vi "Set Position.vi"(0 "LV MDI.lvclass":refnum<class "LV MDI.lvclass">, 5 "Doc UID[]":string[](array[string]), 7 "Position[]":T1[](array[typedef]), 11 "error in (no error)":errorcluster) -> (4 "LV MDI.lvclass":refnum<class "LV MDI.lvclass">, 15 "error out":errorcluster)   [LabVIEW 2016, in "LV MDI.lvclass"]
doc: "Set Position for selected Documents"
uses:
  LV MDI.lvclass
  protected/Postion.ctl
  Document/Document base/Document.lvclass/Document.ctl
  Document/Document base/Document.lvclass
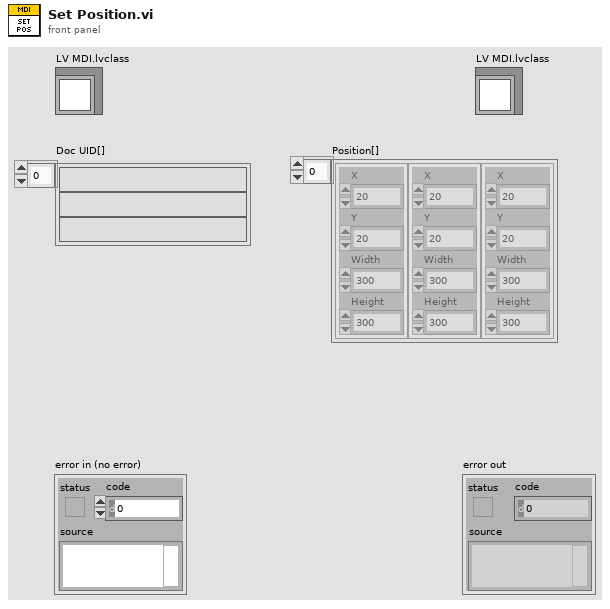
[diagram p1: front panel]
types:
  T1 = typedef "LV MDI.lvclass/Postion.ctl" = cluster{"X":i32, "Y":i32, "Width":i32, "Height":i32}
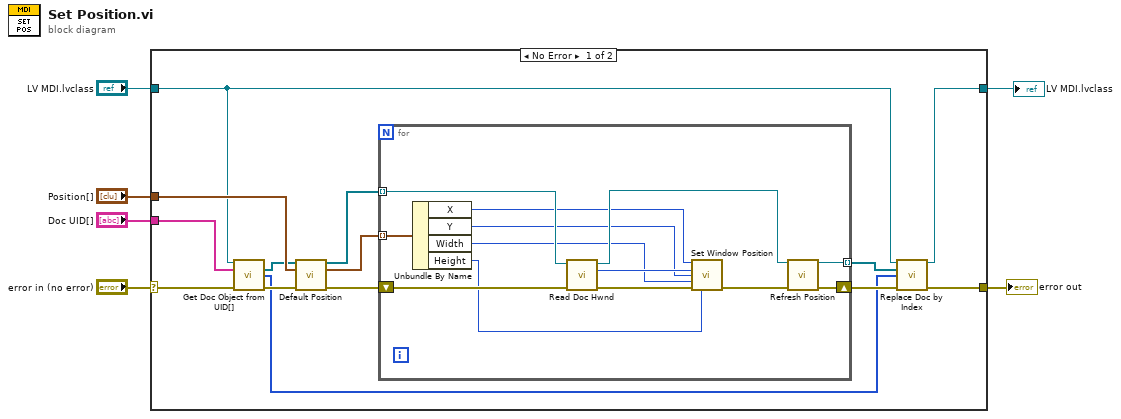
[diagram p0: block diagram]
diagram:
  n1 = case shown="No Error" "error in (no error)" {
    selector: "error in (no error)" -> [w20 w35]
    tunnel: [w11 w35] -> w5
    tunnel: [w10 w34] -> w3
    tunnel: "LV MDI.lvclass" -> [w7 w34]
    tunnel: "Doc UID[]" -> [w19 _]
    tunnel: "Position[]" -> [w16 _]
    frame No Error {
      n2 = call "Get Doc Object from UID[].vi"("LV MDI"=w7, "Doc ÙID[]"=w19, "error in"=w20) -> ("Doc obj[]"=w13:refnum<class "Document.lvclass">[], "Doc index[]"=w8:i32[], "error Out"=w18:errorcluster)  [unwired: 9 in, 1 out]
      n3 = call "Default Position.vi"("Selected Doc[]"=w13, "Position[]"=w16, "error in"=w18) -> ("Selected Doc[]"=w14:refnum<class "Document.lvclass">[], "Position[]"=w15:T1[], "error Out"=w17:errorcluster)  [unwired: 10 in]
      n4 = for {
        shift-right: [w30] -> w12
        shift-left: w17 -> [w33]
        tunnel: w14 -> [w32] mode=indexing
        tunnel: w15 -> [w31] mode=indexing
        tunnel: [w28] -> w9 mode=indexing
        n5 = Unbundle By Name(w31) -> ("X"=w24:i32, "Y"=w22:i32, "Width"=w21:i32, "Height"=w25:i32)
        n6 = call "Read Doc Hwnd.vi"("error in (no error)"=w33, "Document in"=w32) -> ("error out"=w26:errorcluster, "Child Hwnd"=w23:u32, "Document out"=w29:refnum<class "Document.lvclass">)  [unwired: 7 in]
        n7 = call "Set Window Position.vi"("X"=w24, "Hwnd"=w23, "Y"=w22, "Width"=w21, "error in (no error)"=w26, "Height"=w25) -> ("error out"=w27:errorcluster)  [unwired: 9 in]
        n8 = call-dynamic "Refresh Position.vi"("Document in"=w29, "error in (no error)"=w27) -> ("Document out"=w28:refnum<class "Document.lvclass">, "error out"=w30:errorcluster)  [unwired: 12 in]
      }
      n9 = call "Replace Doc by Index.vi"("LV MDI in"=w7, "Doc Class Object[]"=w9, "Doc index[]"=w8, "error in (no error)"=w12) -> ("LV MDI out"=w10:refnum<class "LV MDI.lvclass">, "error out"=w11:errorcluster)  [unwired: 10 in]
    }
    frame Error {
    }
  }
  "error out" <- w5
  "LV MDI.lvclass" <- w3
